vi "sub_getNextValidGuess.vi"(10 "Array":T1[][](array[typedef]), 11 "Queue in":refnum<queue>) -> (2 "guess":T2, 3 "timed out?":bool)   [LabVIEW 2018]
uses:
  guess.ctl
  cell.ctl
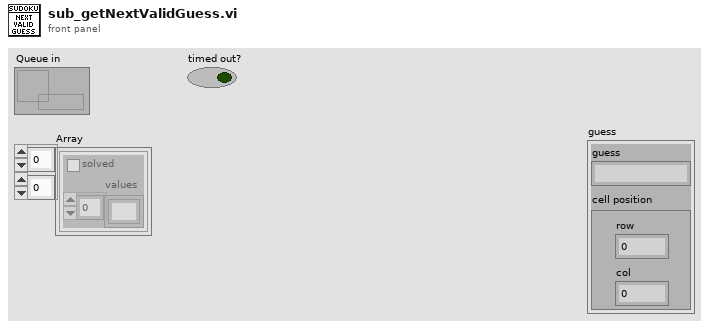
[diagram p1: front panel]
types:
  T1 = typedef "cell.ctl" = cluster{"solved":bool, "values":string[]}
  T2 = typedef "guess.ctl" = cluster{"cell position":cluster{"row":i32, "col":i32}, "guess":string}
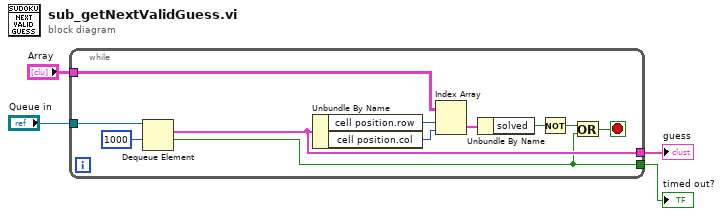
[diagram p0: block diagram]
diagram:
  n1 = while {
    tunnel: "Queue in" -> [w15]
    tunnel: [w6] -> w2
    tunnel: [w13] -> w4
    tunnel: "Array" -> [w12]
    stop <- w5 stop-if-true
    n2 = Dequeue Element(queue=w15, timeout in ms (-1)=1000) -> (element=w13:T2, timed out?=w6:bool)  [unwired: 1 in, 2 out]
    n3 = Unbundle By Name(w13) -> ("cell position.row"=w11:i32, "cell position.col"=w10:i32)
    n4 = Index Array(array=w12, index (row)=w11, index (col)=w10) -> (element=w9:T1)
    n5 = Unbundle By Name(w9) -> ("solved"=w8:bool)
    n6 = Not(x=w8) -> (.not. x?=w7:bool)
    n7 = Or(x=w7, y=w6) -> (x .or. y?=w5:bool)
  }
  "guess" <- w4
  "timed out?" <- w2
